vi "GUI_Scopes_1.0.0.vi"() -> ()   [LabVIEW 2013]
uses:
  <vilib>/Utility/miscctls.llb/LVRectTypeDef.ctl
  Device Drivers/shared/scopeTraceInfo_TypDEf.ctl
  Shared/type definition/trace_TypDef.ctl
  Device Drivers/PXIdigitizer/coupling_Enum_TypDef.ctl
  Device Drivers/PXIdigitizer/impedance_Enum_TypDEf.ctl
panel:
  out "ratio(h)":bool=TRUE
  out "fixsize":bool
  out "Change Ratio":cluster{"X":sgl, "Y":sgl}={"X"=1.6671598, "Y"=0.6151203}
  out "old Panel Bounds":T1={"Left"=105, "Top"=80, "Right"=781, "Bottom"=662}
  in  "shotnumber":i32=354
  in  "Save":bool
  in  "Trigger":bool
  in  "Trig.Delay":dbl
  out "error (h)":bool
  in  "impedance":T2
  in  "Channel":enum16{"Channel1", "Channel2"}(ring)
  in  "probeattenuation":dbl
  out "Channel Selector":string
  in  "channelenabled":enum16{"off", "on"}(ring)
  in  "coupling":T3
  in  "offset":dbl=0.52
  in  "verticalrange":dbl
  in  "scopeTrace.Channel1":T4
  in  "scopeTrace.Channel2":T4
  out "Device Name (h)":string="FakeCam1"
  in  "Main Tap":enum32{"IMAQ", "Network", "Internal", "Array"}(tab)
  out "XY Graph":cluster{dbl, dbl}[](graph)
  out "output waveform":waveform(dbl)[](graph)
  out "local Port":u16=65401
  out "Remote Host":string="192.168.10.157"
  out "port or service name":u16=65400
  in  "timeout ms (slow resp)":i32=500
  in  "reset":bool
  out "image con closed":bool=TRUE
  out "image \nconnection":bool
  out "image con closed 2":bool=TRUE
  out "image \nconnection 2":bool
  out "All Devices (h)":string[](array[string])
  out "fast ID (h)":refnum<k16>
  out "slow ID (h)":refnum<k16>
  out "error out":errorcluster
  out "data connection ID (h)":refnum<k5>
  out "connections (hidden)":variant[](array[variant])=[variant(refnum<k16> refnum), variant(refnum<k16> refnum)]
  in  "time to wait (main loop)":i32=10
  in  "Data String":string="exposure,0.520000\r\ntrigger,off\r\nsave,off\r\ngain,0.000000\r\n"
  out "data out":string="Cam1>>ScanStart>>no error,>>"
  in  "send":bool
  in  "send command":string="ScanStart>>Cam1only.txt"
  out "error 2":bool
  out "error message 2":string
  in  "Local Saving Path":path
  out "stop":bool
  out "error message":string
  out "con ref array":refnum<vi>[](array[refnum])
  out "image connection":bool
  out "data connection ok":bool
  # "Data"
  # "Image"
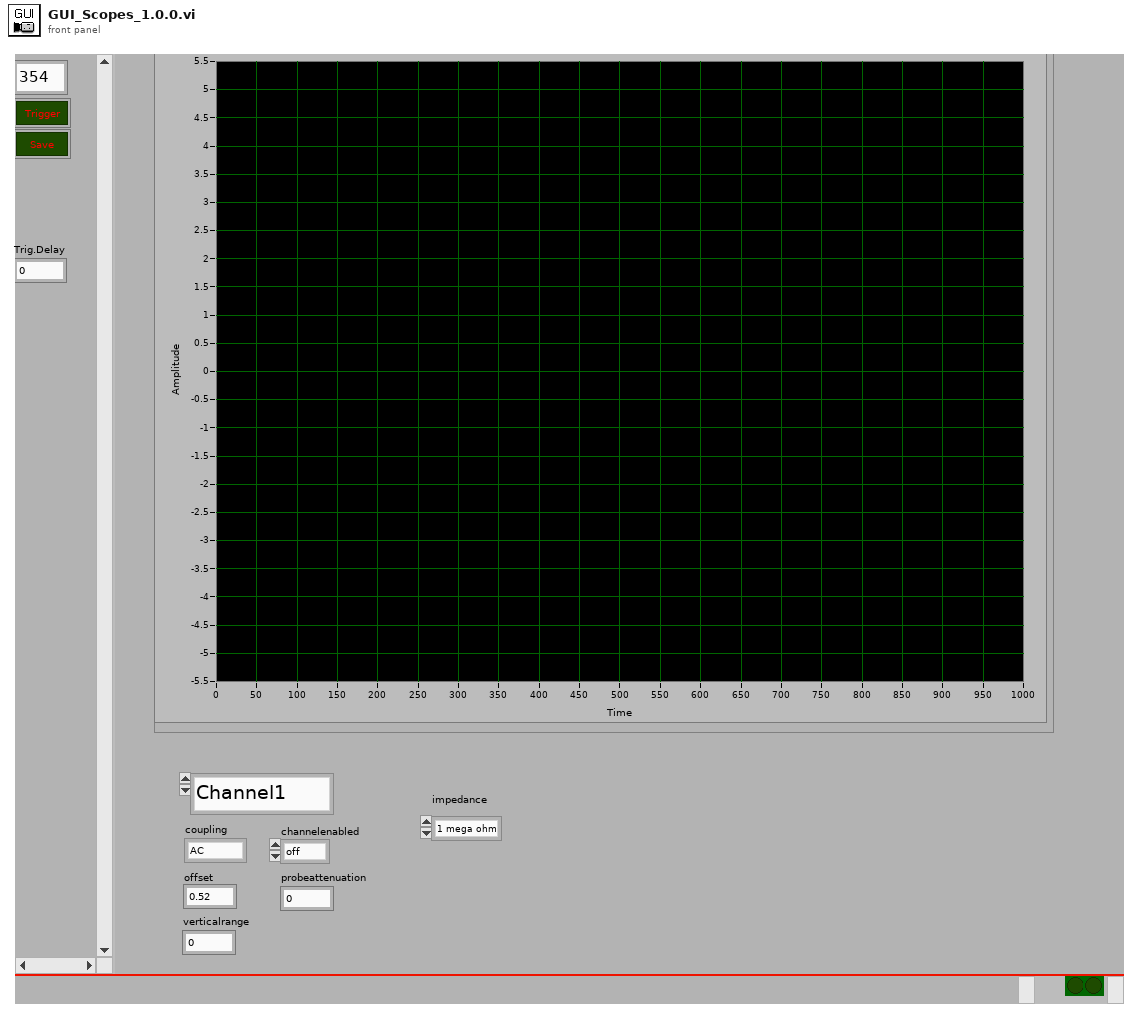
[diagram p1: front panel]
types:
  T1 = typedef "LVRectTypeDef.ctl" = cluster{"Left":i16, "Top":i16, "Right":i16, "Bottom":i16}
  T2 = typedef "impedance_Enum_TypDEf.ctl" = enum16{"1 mega ohm", "<NA>", "50 ohms"}
  T3 = typedef "coupling_Enum_TypDef.ctl" = enum16{"AC", "DC", "Ground"}
  T4 = typedef "trace_TypDef.ctl" = cluster{"info":T5, "wfm":dbl[]}
  T5 = typedef "scopeTraceInfo_TypDEf.ctl" = cluster{"Name":string, "N":dbl, "t0":dbl, "dt":dbl, "offset":dbl, "gain":dbl, "coupling":string, "impedance":string, "range":dbl}
  T6 = typedef "LVBoundsTypeDef.ctl" = cluster{"Width":u32, "Height":u32}
  T7 = typedef "Type Descriptor__ogtk.ctl" = i16[]
  T8 = typedef "Type Descriptor Enumeration__ogtk.ctl" = enum8{"<Null>", "I8", "I16", "I32", "I64", "U8", "U16", "U32", "U64", "SGL", "DBL", "EXT", "CSG", "CDB", "CXT", "0x0F", "0x10", "0x11", "0x12", "0x13", "0x14", "Enum U8", "Enum U16", "Enum U32", "Enum U64", "SGL PQ", "DBL PQ", "EXT PQ", "CSG PQ", "CDB PQ", "CXT PQ", "0x1F", "0x20", "Boolean", "0x22", "0x23", "0x24", "0x25", "0x26", "0x27", "0x28", "0x29", "0x2A", "0x2B", "0x2C", "0x2D", "0x2E", "0x2F", "String", "0x31", "Path", "Pict", "0x34", "0x35", "0x36", "DAQ", "0x38", "0x39", "0x3A", "0x3B", "0x3C", "0x3D", "0x3E", "0x3F", "Array", "0x41", "0x42", "0x43", "0x44", "0x45", "0x46", "0x47", "0x48", "0x49", "0x4A", "0x4B", "0x4C", "0x4D", "0x4E", "0x4F", "Cluster", "0x51", "0x52", "Variant", "Waveform", "0x55", "0x56", "0x57", "0x58", "0x59", "0x5A", "0x5B", "0x5C", "0x5D", "0x5E", "0x5F", "0x60", "0x61", "0x62", "0x63", "0x64", "0x65", "0x66", "0x67", "0x68", "0x69", "0x6A", "0x6B", "0x6C", "0x6D", "0x6E", "0x6F", "Refnum"}
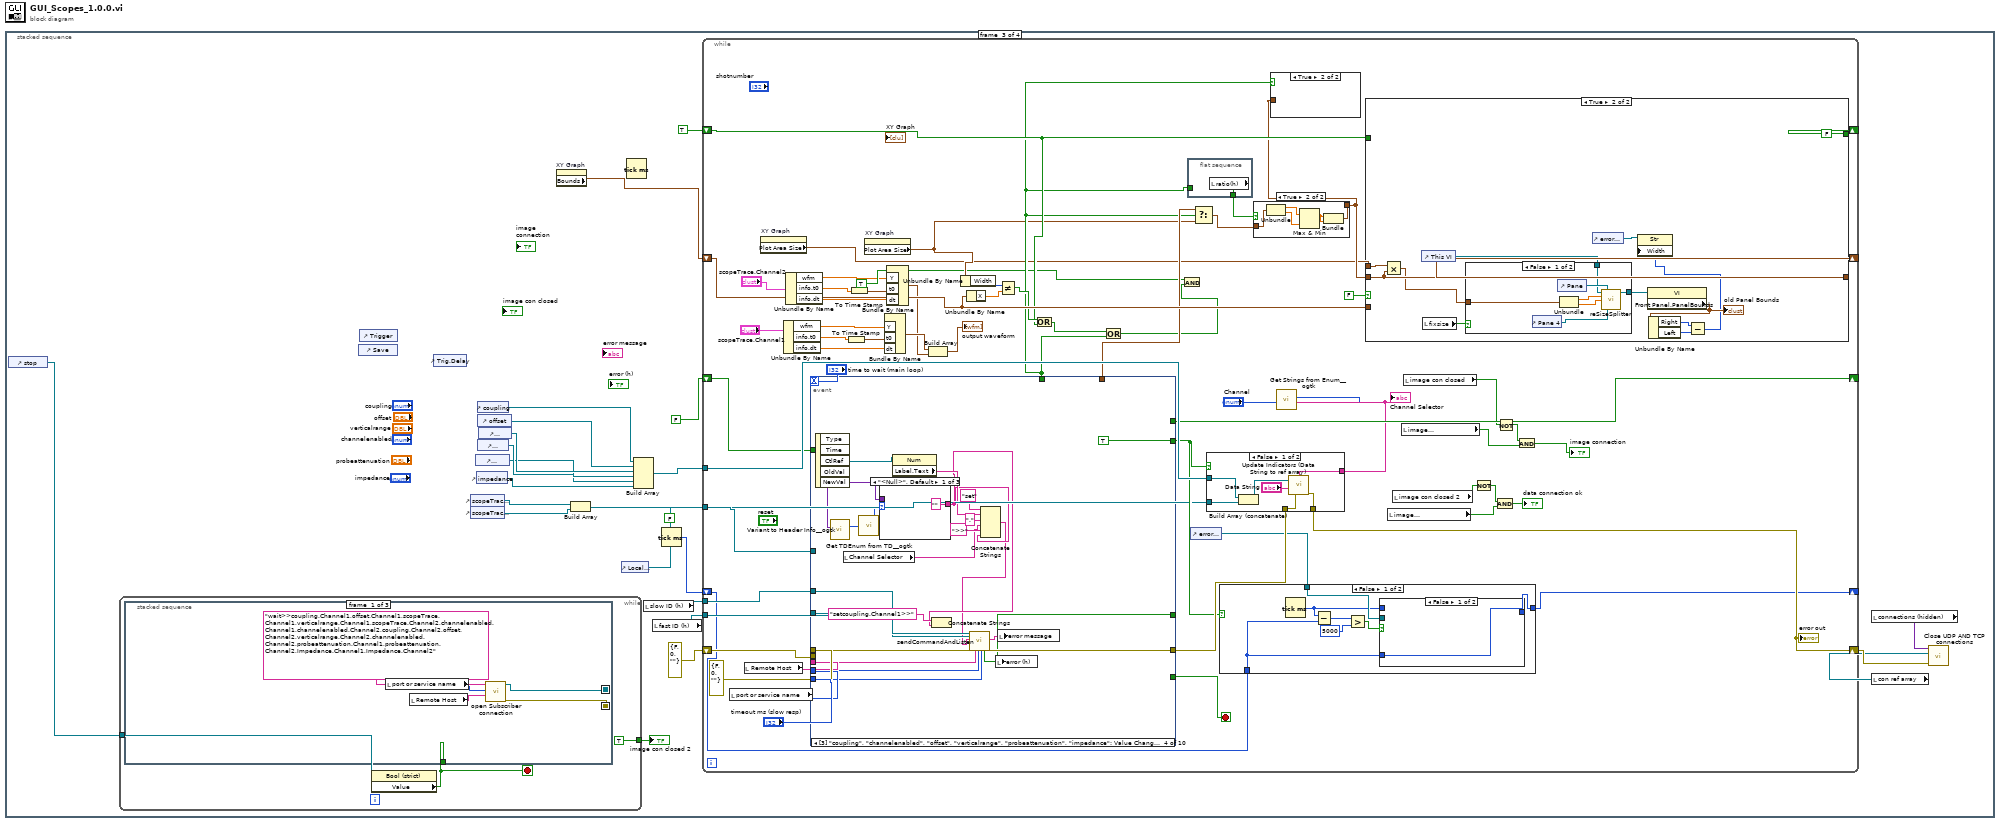
[diagram p0: block diagram]
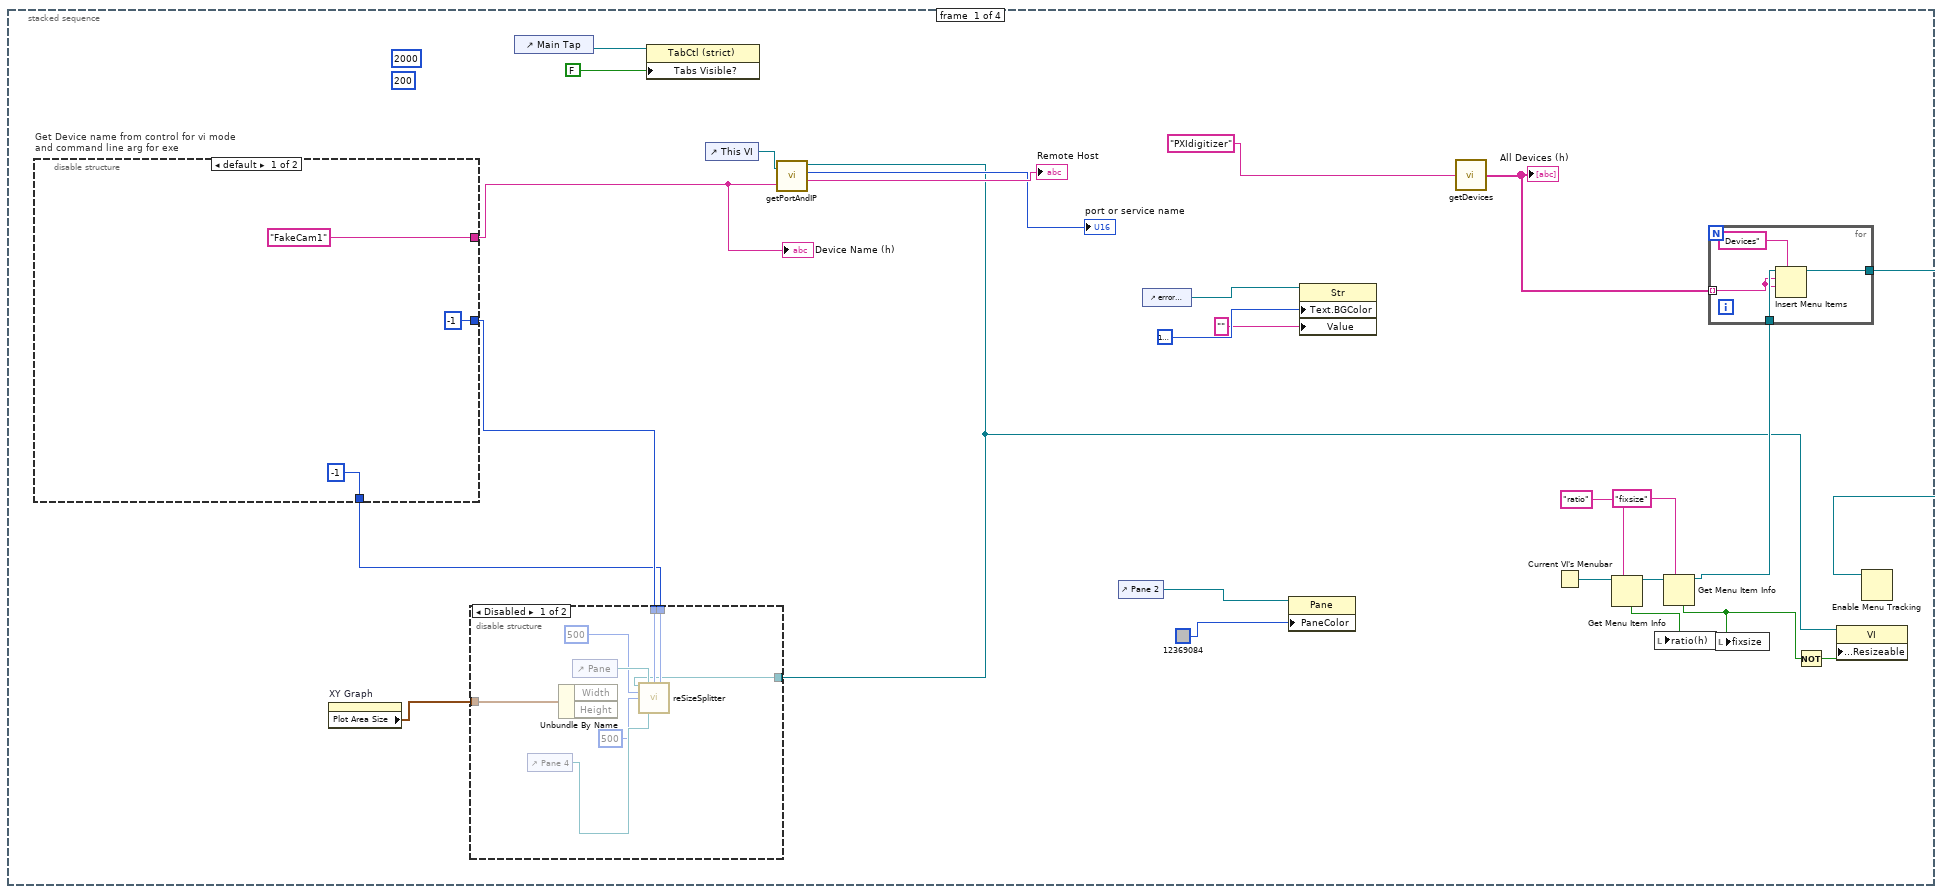
[diagram p2: hidden frame]
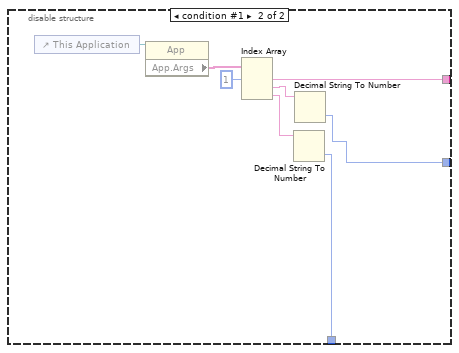
[diagram p4: hidden frame]
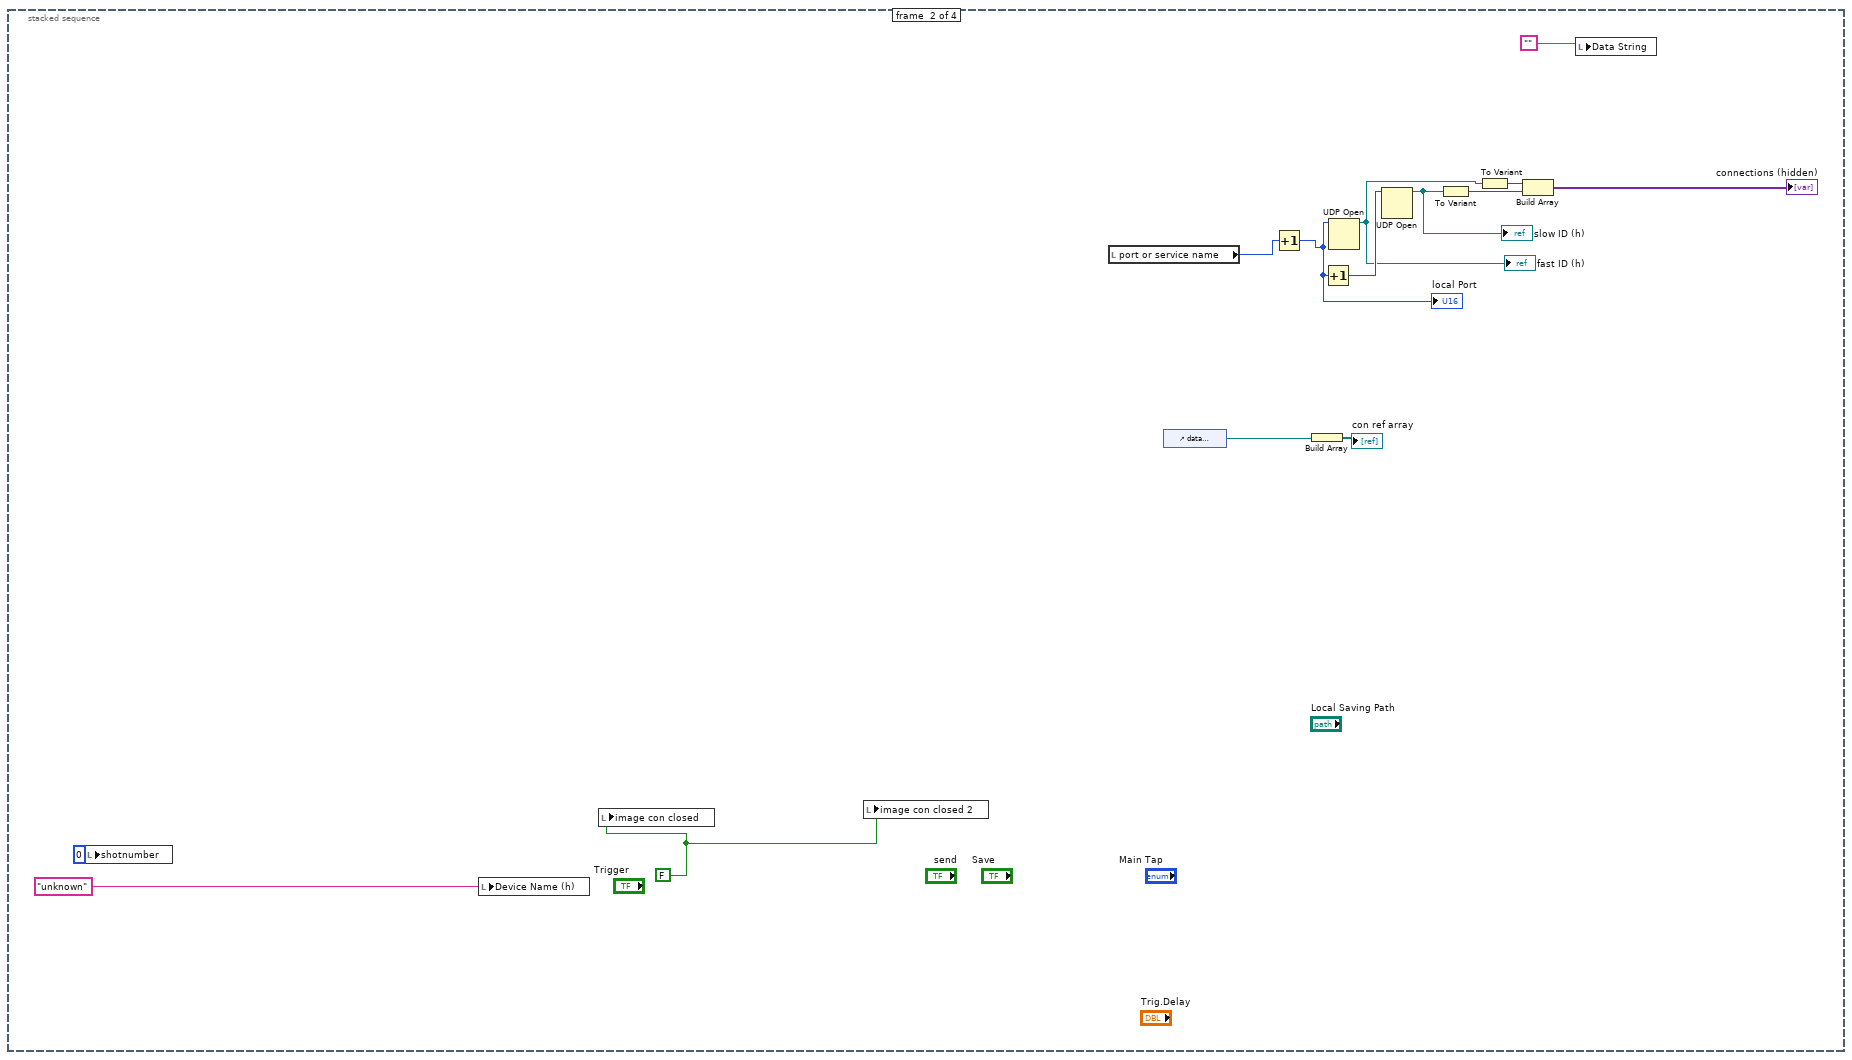
[diagram p5: hidden frame]
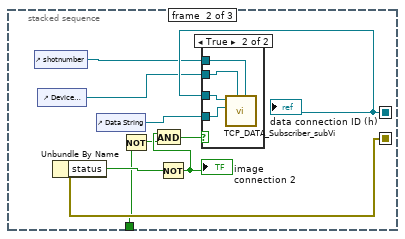
[diagram p6: hidden frame]
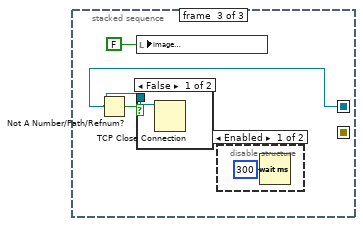
[diagram p8: hidden frame]
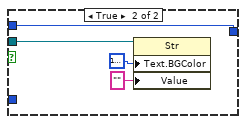
[diagram p11: hidden frame]
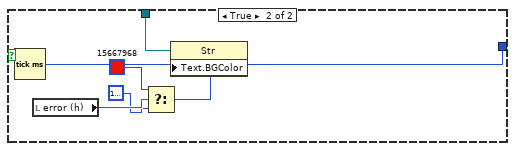
[diagram p12: hidden frame]
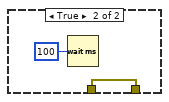
[diagram p17: hidden frame]
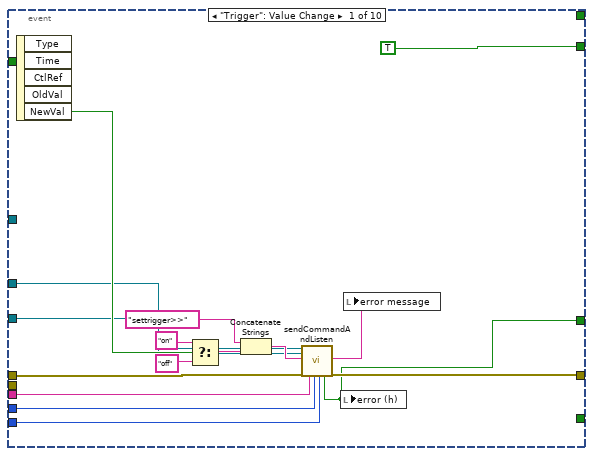
[diagram p18: hidden frame]
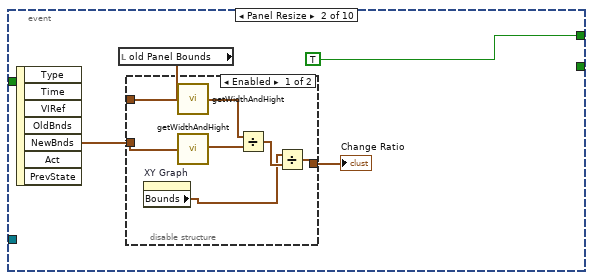
[diagram p19: hidden frame]
diagram:
  n1 = stacked-sequence {
    frame #0 {
      (unwired) i16 2000 ("Left")
      (unwired) i16 200 ("Top")
      n2 = disable-structure "Get Device name from control for vi mode\nand command line arg for exe" shown="default" {
        disable-tunnel: ["FakeCam1" ("Device Name for vi mode") w46] -> w5
        disable-tunnel: [i16 -1 ("left") w43] -> w19
        disable-tunnel: [i16 -1 ("left") w42] -> w18
        frame condition #0 (active) {
        }
        frame condition #1 {
          n3 = control-ref of="This Application"() -> (w49:refnum<vi>)
          n4 = property class="App"(reference=w49) -> ("App.Args"=w48:string[])  [unwired: 1 in, 2 out]
          n5 = Index Array(array=w48, index #1=1 ("index")) -> (element #1=w46:string, element #2=w45:string, element #3=w44:string)  [unwired: 2 in]
          n6 = Decimal String To Number(string=w44) -> (number=w42:i32)  [unwired: 2 in, 1 out]
          n7 = Decimal String To Number(string=w45) -> (number=w43:i32)  [unwired: 2 in, 1 out]
        }
      }
      "Device Name (h)" <- w5
      n8 = property on="XY Graph" class="XYGraph (strict)"() -> ("Plot Area Size"=w1:T6)  [unwired: 2 in, 2 out]
      n9 = control-ref of="Main Tap"() -> (w26:refnum<vi>)
      n10 = property class="TabCtl (strict)"(reference=w26, "Tabs Visible?"=FALSE) -> ()  [unwired: 1 in, 2 out]
      n11 = control-ref of="This VI"() -> (w4:refnum<vi>)
      n12 = call "getPortAndIP.vi"("This Vi"=w4, "Device Name"=w5) -> ("reference out"=w3:refnum<vi>, "port or service name"=→"port or service name":u16, "Remote Host"=→"Remote Host":string)  [unwired: 1 in]
      n13 = disable-structure shown="Disabled" {
        disable-tunnel: w19 -> [w33 _]
        disable-tunnel: w18 -> [w32 _]
        disable-tunnel: w3 -> [w30 _]
        disable-tunnel: w1 -> [w29 _]
        frame Disabled {
          n14 = control-ref of="Pane 4"() -> (w31:refnum<vi>)
          n15 = Unbundle By Name(w29) -> ()  [unwired: 2 out]
          n16 = control-ref of="Pane"() -> (w34:refnum<vi>)
          n17 = call "reSizeSplitter.vi"("this vi"=w30, "pane"=w34, "left"=w33, "top"=w32, "Width"=u32 500, "Height"=u32 500, "pane2"=w31) -> ()  [unwired: 8 in, 1 out]
        }
        frame Enabled {
        }
      }
      n18 = control-ref of="Pane 2"() -> (w12:refnum<vi>)
      n19 = control-ref of="error message"() -> (w14:refnum<vi>)
      n20 = property class="Pane"(reference=w12, "PaneColor"=u32 12369084) -> ()  [unwired: 1 in, 2 out]
      n21 = property class="Str"(reference=w14, "Text.BGColor"=u32 16777238, "Value"="") -> ()  [unwired: 1 in, 2 out]
      n22 = call "getDevices.vi"("Device Class"="PXIdigitizer") -> ("All Devices"=w8:string[])
      "All Devices (h)" <- w8
      n23 = Current VI's Menubar() -> (w23:refnum<k9>)
      n24 = Get Menu Item Info(7:"ratio" ("item tag"), 11:w23) -> (3:w21:refnum<k9>, 4:w22:bool)  [unwired: 1 in, 5 out]
      n25 = local write "ratio(h)"(w22) -> ()
      n26 = Get Menu Item Info(7:"fixsize" ("item tag"), 11:w21) -> (3:w10:refnum<k9>, 4:w16:bool)  [unwired: 1 in, 5 out]
      n27 = for {
        tunnel: w10 -> [w38]
        tunnel: [w37] -> w9
        tunnel: w8 -> [w35] mode=indexing
        n28 = Insert Menu Items(5:"Devices" ("menu tag"), 7:w35, 8:w35, 9:w38) -> (3:w37:refnum<k9>)  [unwired: 2 in, 2 out]
      }
      n29 = local write "fixsize"(w16) -> ()
      n30 = Not(x=w16) -> (.not. x?=w17:bool)
      n31 = property class="VI"(reference=w3, "Front Panel.Resizeable"=w17) -> ()  [unwired: 1 in, 2 out]
      n32 = Enable Menu Tracking(4:w9) -> ()  [unwired: 2 in, 2 out]
    }
    frame #1 {
      w59 = FALSE ("new Device Data")
      n33 = local write "shotnumber"(0 ("shotnumber")) -> ()
      n34 = local write "Device Name (h)"("unknown" ("Device Name")) -> ()
      n35 = local write "image con closed"(w59) -> ()
      n36 = local write "image con closed 2"(w59) -> ()
      n37 = local read "port or service name"() -> (w55:u16)
      n38 = control-ref of="data connection ID (h)"() -> (w63:refnum<vi>)
      n39 = Increment(x=w55) -> (x+1=w52:u16)
      "local Port" <- w52
      n40 = Build Array(w63) -> (→"con ref array":refnum<vi>[])
      n41 = Increment(x=w52) -> (x+1=w56:u16)
      n42 = UDP Open(11:w52) -> (port=w53:refnum<k16>)  [unwired: 4 in, 2 out]
      "fast ID (h)" <- w53
      n43 = UDP Open(11:w56) -> (port=w54:refnum<k16>)  [unwired: 4 in, 2 out]
      "slow ID (h)" <- w54
      n44 = To Variant(anything=w54) -> (Variant=w58:variant)
      n45 = To Variant(anything=w53) -> (Variant=w57:variant)
      n46 = Build Array(w57, w58) -> (→"connections (hidden)":variant[])
      n47 = local write "Data String"("") -> ()
    }
    frame #2 {
      (unwired) FALSE
      n48 = control-ref of="stop"() -> (w79:refnum<vi>)
      n49 = while {
        tunnel: [TRUE] -> w80
        tunnel: w79 -> [w88]
        stop <- w87 stop-if-true
        n50 = property class="Bool (strict)"(reference=w88) -> ("Value"=w87:bool)  [unwired: 1 in, 2 out]
        n51 = stacked-sequence {
          seq-local: [w91 _ _] -> [_ w103 w110]
          seq-local: [w90 _ _] -> [_ w102 _]
          tunnel: w87 -> [_ w96 _]
          frame #0 {
            n52 = local read "port or service name"() -> (w93:u16)
            n53 = local read "Remote Host"() -> (w92:string)
            n54 = call "open Subscriber connection.vi"("Machine"=w92, "Port"=w93, "Subscriber list"="wait>>coupling.Channel1,offset.Channel1,scopeTrace.Channel1,verticalrange.Channel1,scopeTrace.Channel2,channelenabled.Channel1,channelenabled.Channel2,coupling.Channel2,offset.Channel2,verticalrange.Channel2,channelenabled.Channel2,probeattenuation.Channel1,probeattenuation.Channel2,Impedance.Channel1,Impedance.Channel2" ("Subscriber list 2")) -> ("error out"=w90:errorcluster, "connection ID"=w91:refnum<k5>)  [unwired: 3 in]
          }
          frame #1 {
            n55 = control-ref of="shotnumber"() -> (w101:refnum<vi>)
            n56 = control-ref of="Device Name (h)"() -> (w100:refnum<vi>)
            n57 = Unbundle By Name(w102) -> ("status"=w99:bool)
            n58 = control-ref of="Data String"() -> (w104:refnum<vi>)
            n59 = Not(x=w96) -> (.not. x?=w97:bool)
            n60 = Not(x=w99) -> (.not. x?=w98:bool)
            "image \nconnection 2" <- w98
            n61 = And(x=w98, y=w97) -> (x .and. y?=w95:bool)
            n62 = case shown="True" w95 {
              tunnel: w104 -> [_ w108]
              tunnel: w103 -> [_ w107]
              tunnel: w101 -> [_ w106]
              tunnel: w100 -> [_ w105]
              frame False {
              }
              frame True {
                n63 = call "TCP_DATA_Subscriber_subVi.vi"("shot number"=w106, "whatamI"=w105, 10:w108, "connection ID"=w107) -> ()  [unwired: 7 in, 1 out]
              }
            }
            "data connection ID (h)" <- w103
          }
          frame #2 {
            n64 = Not A Number/Path/Refnum?(number/path/refnum=w110) -> (NaN/Path/Refnum?=w111:bool)
            n65 = local write "image \nconnection 2"(FALSE ("status 2")) -> ()
            n66 = case shown="False" w111 {
              tunnel: w110 -> [w113 _]
              frame False {
                n67 = TCP Close Connection(connection ID=w113) -> ()  [unwired: 2 in, 2 out]
              }
              frame True {
              }
            }
            n68 = disable-structure shown="Enabled" {
              frame Enabled {
                n69 = Wait (ms)(milliseconds to wait=u32 300 ("millisecond multiple")) -> ()  [unwired: 1 out]
              }
              frame Disabled {
              }
            }
          }
        }
      }
      "image con closed 2" <- w80
      n70 = control-ref of="Save"() -> ()  [unwired: 1 out]
      n71 = control-ref of="Trigger"() -> ()  [unwired: 1 out]
      n72 = control-ref of="Trig.Delay"() -> ()  [unwired: 1 out]
      n73 = control-ref of="scopeTrace.Channel1"() -> (w68:refnum<vi>)
      n74 = control-ref of="scopeTrace.Channel2"() -> (w67:refnum<vi>)
      n75 = control-ref of="probeattenuation"() -> (w65:refnum<vi>)
      n76 = control-ref of="impedance"() -> (w64:refnum<vi>)
      n77 = control-ref of="coupling"() -> (w71:refnum<vi>)
      n78 = control-ref of="offset"() -> (w72:refnum<vi>)
      n79 = control-ref of="channelenabled"() -> (w69:refnum<vi>)
      n80 = control-ref of="verticalrange"() -> (w70:refnum<vi>)
      n81 = property on="XY Graph" class="XYGraph (strict)"() -> ("Bounds"=w74:T6)  [unwired: 2 in, 2 out]
      n82 = Build Array(w68, w67) -> (w66:refnum<vi>[])
      n83 = control-ref of="Local Saving Path"() -> (w75:refnum<vi>)
      n84 = Tick Count (ms)() -> ()  [unwired: 1 out]
      n85 = Build Array(w71, w72, w70, w69, w65, w64) -> (w73:refnum<vi>[])
      n86 = local read "slow ID (h)"() -> (w84:refnum<k16>)
      n87 = local read "fast ID (h)"() -> (w85:refnum<k16>)
      n88 = Tick Count (ms)() -> (millisecond timer value=w76:u32)
      n89 = while {
        tunnel: w85 -> [w167]
        shift-right: [w164] -> w83
        shift-left: errorcluster {"status"=FALSE, "code"=0, "source"=""} ("error out") -> [w170]
        tunnel: w84 -> [w166]
        tunnel: w73 -> [w172]
        shift-right: [w163] -> _
        shift-left: w74 -> [w162]
        shift-right: [w156] -> _
        shift-left: FALSE -> [w157]
        shift-right: [w155] -> _
        shift-left: TRUE -> [w154]
        shift-right: [w138] -> _
        shift-left: w76 -> [w137]
        tunnel: w75 -> [w134]
        tunnel: w66 -> [w116]
        stop <- w159 stop-if-true
        n90 = local read "port or service name"() -> (w168:u16)
        n91 = local read "Remote Host"() -> (w169:string)
        n92 = property on="XY Graph" class="XYGraph (strict)"() -> ("Plot Area Size"=w132:T6)  [unwired: 2 in, 2 out]
        n93 = Unbundle By Name("scopeTrace.Channel1") -> ("wfm"=w128:dbl[], "info.t0"=w127:dbl, "info.dt"=w125:dbl)
        n94 = Unbundle By Name("scopeTrace.Channel2") -> ("wfm"=w119:dbl[], "info.t0"=w120:dbl, "info.dt"=w122:dbl)
        n95 = event shown="[3] \"coupling\", \"channelenabled\", \"offset\", \"verticalrange\", \"probeattenuation\", \"impedance\": Value Change" {
          selector: _ -> [_ _ _ _ _ _ _ _ _ _]
          dyn-events: _ -> [_ _ _ _ _ _ _ _ _ _]
          timeout: "time to wait (main loop)" -> [_ _ _ _ _ _ _ _ _ _]
          tunnel: w167 -> [w236 _ _ w281 w298 w314 w326 w343 _ _]
          tunnel: [w234 _ _ w279 w296 w312 w323 w341 w349 _] -> w165
          tunnel: errorcluster {"status"=FALSE, "code"=0, "source"=""} ("error out") -> [w235 _ _ w280 w297 w313 w324 w342 _ _]
          tunnel: w169 -> [w239 _ _ w278 w295 w311 w327 w340 _ _]
          tunnel: w168 -> [w240 _ _ w277 w294 w310 w322 w339 _ _]
          tunnel: "timeout ms (slow resp)" -> [w241 _ _ w276 w293 w309 w321 w338 _ _]
          tunnel: w166 -> [w237 _ _ w282 w299 w315 w325 w344 _ _]
          tunnel: w170 -> [_ _ _ _ _ _ _ _ w349 _]
          tunnel: [TRUE _ _ TRUE TRUE TRUE TRUE TRUE _ _] -> w135
          tunnel: [_ _ _ _ _ _ _ _ _ w355] -> w159
          tunnel: [_ _ _ _ _ _ _ _ w348 w352] -> w147
          tunnel: w157 -> [_ _ _ _ _ _ _ _ w348 _]
          tunnel: [_ TRUE _ _ _ _ _ _ _ _] -> w156
          tunnel: [_ _ _ _ _ _ _ _ w347 _] -> w151
          tunnel: [w231 _ _ w273 w290 w304 w318 w334 _ _] -> _
          tunnel: w134 -> [_ _ _ _ _ _ _ _ _ w350]
          event "Trigger": Value Change {
            n96 = event-data() -> ("NewVal"=w246:bool)  [unwired: 1 in, 4 out]
            n97 = Select(t="on", s=w246, f="off") -> (s? t:f=w242:string)
            n98 = Concatenate Strings("settrigger>>" ("data in"), w242) -> (w238:string)
            n99 = call "sendCommandAndListen.vi"(0:w237, 1:w236, "command in"=w238, "error in"=w235, "Remote Host"=w239, "port or service name"=w240, "timeout ms (100)"=w241) -> ("error"=w231:bool, "error message"=w233:string, "error out"=w234:errorcluster)  [unwired: 5 in, 5 out]
            n100 = local write "error (h)"(w231) -> ()
            n101 = local write "error message"(w233) -> ()
          }
          event Panel Resize {
            n102 = event-data() -> ("NewBnds"=w250:T1)  [unwired: 1 in, 6 out]
            n103 = local read "old Panel Bounds"() -> (w248:T1)
            n104 = disable-structure shown="Enabled" {
              disable-tunnel: w250 -> [w257 _]
              disable-tunnel: w248 -> [w253 _]
              disable-tunnel: [w252 _] -> w247
              frame Enabled {
                n105 = property on="XY Graph" class="XYGraph (strict)"() -> ("Bounds"=w251:T6)  [unwired: 2 in, 2 out]
                n106 = call "getWidthAndHight.vi"("OldBnds"=w253) -> ("output cluster"=w256:cluster{"X":sgl, "Y":sgl})
                n107 = call "getWidthAndHight.vi"("OldBnds"=w257) -> ("output cluster"=w255:cluster{"X":sgl, "Y":sgl})
                n108 = Divide(x=w256, y=w255) -> (x/y=w254:cluster{"X":sgl, "Y":sgl})
                n109 = Divide(x=w251, y=w254) -> (x/y=w252:cluster{sgl, sgl})
              }
              frame Disabled {
              }
            }
            "Change Ratio" <- w247
          }
          event "reset": Value Change {
            n110 = event-data() -> ()  [unwired: 1 in, 5 out]
            n111 = flat-sequence {
              frame #0 {
                n112 = local read "con ref array"() -> (w259:refnum<vi>[])
                n113 = call "Close UDP AND TCP connections.vi"("appended array 2"=w259) -> ()  [unwired: 7 in]
              }
              frame #1 {
                n114 = Wait (ms)(milliseconds to wait=u32 1000) -> ()  [unwired: 1 out]
              }
            }
            n115 = local write "reset"(FALSE ("reset")) -> ()
          }
          event "channelenabled", "offset", "verticalrange", "probeattenuation": Value Change {
            n116 = event-data() -> ("CtlRef"=w272:refnum<vi>, "NewVal"=w263:variant)  [unwired: 1 in, 3 out]
            n117 = call <userlib>:"Variant to Header Info__ogtk.vi"("Variant"=w263) -> ("Type Descriptor"=w262:T7)  [unwired: 3 in, 2 out]
            n118 = local read "Channel Selector"() -> (w264:string)
            n119 = call <userlib>:"Get TDEnum from TD__ogtk.vi"("Type Descriptor"=w262) -> ("Type Descriptor Enumeration"=w261:T8)  [unwired: 4 in]
            n120 = case shown="\"<Null>\", Default" w261 {
              tunnel: ["" ("String Value") w285 w286] -> w266
              tunnel: w263 -> [_ w284 w289]
              frame "<Null>", Default {
              }
              frame "Enum U16" {
                n121 = call <userlib>:"Get Strings from Enum__ogtk.vi"("Enum"=w284) -> ("String Value"=w285:string)  [unwired: 7 in, 3 out]
              }
              frame "I8".."CXT" {
                n122 = Variant To Data(type=0.0, Variant=w289) -> (data=w287:dbl)  [unwired: 1 in, 1 out]
                n123 = Number To Fractional String(number=w287) -> (F-format string=w286:string)  [unwired: 3 in]
              }
            }
            n124 = property class="Num"(reference=w272) -> ("Label.Text"=w270:string)  [unwired: 1 in, 2 out]
            n125 = Concatenate Strings("setcoupling.Channel1>>" ("data in"), w266) -> ()  [unwired: 1 out]
            n126 = Concatenate Strings("set", w270, "." ("string"), w264, ">>" ("string"), w266) -> (w265:string)
            n127 = call "sendCommandAndListen.vi"(0:w282, 1:w281, "command in"=w265, "error in"=w280, "Remote Host"=w278, "port or service name"=w277, "timeout ms (100)"=w276) -> ("error"=w273:bool, "error message"=w275:string, "error out"=w279:errorcluster)  [unwired: 5 in, 5 out]
            n128 = local write "error (h)"(w273) -> ()
            n129 = local write "error message"(w275) -> ()
          }
          event "Trig.Delay": Value Change {
            n130 = event-data() -> ("NewVal"=w301:dbl)  [unwired: 1 in, 4 out]
            n131 = Number To Fractional String(number=w301) -> (F-format string=w302:string)  [unwired: 3 in]
            n132 = Concatenate Strings("settriggerdelay>>" ("data in"), w302) -> (w300:string)
            n133 = call "sendCommandAndListen.vi"(0:w299, 1:w298, "command in"=w300, "error in"=w297, "Remote Host"=w295, "port or service name"=w294, "timeout ms (100)"=w293) -> ("error"=w290:bool, "error message"=w292:string, "error out"=w296:errorcluster)  [unwired: 5 in, 5 out]
            n134 = local write "error (h)"(w290) -> ()
            n135 = local write "error message"(w292) -> ()
          }
          event "Local Saving Path": Value Change {
            n136 = event-data() -> ("NewVal"=w306:path)  [unwired: 1 in, 4 out]
            n137 = Path To String(path=w306) -> (string=w305:string)
            n138 = Concatenate Strings("setlocalsavingpath>>" ("data in"), w305) -> (w316:string)
            n139 = call "sendCommandAndListen.vi"(0:w315, 1:w314, "command in"=w316, "error in"=w313, "Remote Host"=w311, "port or service name"=w310, "timeout ms (100)"=w309) -> ("error"=w304:bool, "error message"=w308:string, "error out"=w312:errorcluster)  [unwired: 5 in, 5 out]
            n140 = local write "error (h)"(w304) -> ()
            n141 = local write "error message"(w308) -> ()
          }
          event "Save": Value Change {
            n142 = event-data() -> ("NewVal"=w333:bool)  [unwired: 1 in, 4 out]
            n143 = Select(t="on", s=w333, f="off") -> (s? t:f=w329:string)
            n144 = Concatenate Strings("setsave>>" ("data in"), w329) -> (w328:string)
            n145 = call "sendCommandAndListen.vi"(0:w325, 1:w326, "command in"=w328, "error in"=w324, "Remote Host"=w327, "port or service name"=w322, "timeout ms (100)"=w321) -> ("error"=w318:bool, "error message"=w320:string, "error out"=w323:errorcluster)  [unwired: 5 in, 5 out]
            n146 = local write "error (h)"(w318) -> ()
            n147 = local write "error message"(w320) -> ()
          }
          event "send": Value Change {
            n148 = event-data() -> ()  [unwired: 1 in, 5 out]
            n149 = local write "send"(FALSE ("sent")) -> ()
            n150 = call "sendCommandAndListen.vi"(0:w344, 1:w343, "command in"="send command", "error in"=w342, "Remote Host"=w340, "port or service name"=w339, "timeout ms (100)"=w338) -> ("error"=w334:bool, "error message"=→"error message 2":string, "data out"=→"data out":string, "error out"=w341:errorcluster)  [unwired: 5 in, 4 out]
            "error 2" <- w334
          }
          event Timeout {
            n151 = event-data() -> ()  [unwired: 1 in, 2 out]
            n152 = local read "Change Ratio"() -> (w347:cluster{"X":sgl, "Y":sgl})
          }
          event Menu Selection (User) {
            n153 = event-data() -> ("MenuRef"=w351:refnum<k9>, "ItemTag"=w353:string)  [unwired: 1 in, 3 out]
            n154 = Equal?(x="Exit", y=w353) -> (x = y?=w355:bool)
            "stop" <- w355
            n155 = property on="Main Tap" class="TabCtl (strict)"() -> ("Value"=w357:enum32{"IMAQ", "Network", "Internal", "Array"})  [unwired: 2 in, 2 out]
            n156 = case shown="False" w355 {
              tunnel: w357 -> [w410 _]
              tunnel: w353 -> [w409 _]
              tunnel: [w406 errorcluster {"status"=FALSE, "code"=0, "source"=""} ("error out")] -> w354
              frame False {
                n157 = call <userlib>:"Set Enum String Value__ogtk.vi"("String Value"=w409, "Default Enum Value"=w410) -> ("error out"=w408:errorcluster, "Enum"=w412:variant)  [unwired: 8 in]
                n158 = Variant To Data(error in=w408, type=w410, Variant=w412) -> (data=w411:enum32{"IMAQ", "Network", "Internal", "Array"}, error out=w407:errorcluster)
                n159 = property on="Main Tap" class="TabCtl (strict)"(error in=w407, "Value"=w411) -> (error out=w406:errorcluster)  [unwired: 1 in, 1 out]
              }
              frame True {
              }
            }
            n160 = case shown="Error" w354 {
              tunnel: w351 -> [_ w362]
              tunnel: w353 -> [_ w366]
              tunnel: [_ w367] -> w352
              tunnel: w350 -> [_ w360]
              frame No Error {
              }
              frame Error {
                n161 = local read "All Devices (h)"() -> (w364:string[])
                n162 = Get Menu Item Info(7:w366, 11:w362) -> (0:w363:errorcluster, 2:w369:string, 4:w370:bool)  [unwired: 1 in, 4 out]
                n163 = Not(x=w370) -> (.not. x?=w368:bool)
                n164 = Search 1D Array(1D array=w364, element=w366) -> (index of element=w365:i32)  [unwired: 1 in]
                n165 = Greater Or Equal To 0?(x=w365) -> (x >= 0?=w361:bool)
                n166 = case shown="True" w361 {
                  tunnel: w364 -> [_ w374]
                  tunnel: w363 -> [_ _]
                  tunnel: w362 -> [w371 w373]
                  tunnel: [w371 w372] -> w359
                  frame False {
                  }
                  frame True {
                    n167 = for {
                      tunnel: w374 -> [w378] mode=indexing
                      tunnel: w373 -> [w376]
                      tunnel: [w375] -> w372
                      n168 = Set Menu Item Info(6:FALSE ("checked"), 7:w378, 11:w376) -> (3:w375:refnum<k9>)  [unwired: 4 in, 1 out]
                    }
                  }
                }
                n169 = case shown="\"clear\"" w366 {
                  selector: w366 -> [_ w384 _ _ _ _]
                  tunnel: w368 -> [w379 w382 w393 _ _ _]
                  tunnel: [_ _ TRUE _ _ _] -> w367
                  tunnel: w361 -> [_ w385 _ _ _ _]
                  tunnel: w360 -> [_ _ _ w399 _ _]
                  tunnel: [w379 w383 w393 _ _ _] -> w358
                  frame "fixsize" {
                    n170 = control-ref of="This VI"() -> (w381:refnum<vi>)
                    n171 = Not(x=w379) -> (.not. x?=w380:bool)
                    n172 = property class="VI"(reference=w381, "Front Panel.Resizeable"=w380) -> ()  [unwired: 1 in, 2 out]
                    "fixsize" <- w379
                  }
                  frame Default {
                    n173 = case shown="True" w385 {
                      tunnel: w384 -> [_ w392]
                      tunnel: [_ w386] -> w383
                      tunnel: w382 -> [_ w386]
                      frame False {
                      }
                      frame True {
                        n174 = control-ref of="This VI"() -> (w391:refnum<vi>)
                        n175 = control-ref of="reset"() -> (w388:refnum<vi>)
                        n176 = call "getPortAndIP.vi"("This Vi"=w391, "Device Name"=w392) -> ("port or service name"=w389:u16, "Remote Host"=w390:string)  [unwired: 1 in, 1 out]
                        n177 = local write "port or service name"(w389) -> ()
                        n178 = local write "Remote Host"(w390) -> ()
                        n179 = property class="Bool (strict)"(reference=w388, "Val(Sgnl)"=TRUE ("Value (Signaling)")) -> ()  [unwired: 1 in, 2 out]
                      }
                    }
                  }
                  frame "ratio" {
                    "ratio(h)" <- w393
                  }
                  frame "Local Saving Path" {
                    n180 = property class="Path"(reference=w399) -> (reference out=w397:refnum<vi>, "Value"=w398:path)  [unwired: 1 in, 1 out]
                    n181 = call "changePath.vi"("Local Saving in (h)"=w398) -> ("change (h)"=w396:bool, "Local Saving out (h)"=w395:path)  [unwired: 9 in]
                    n182 = case shown="True" w396 {
                      tunnel: w397 -> [_ w401]
                      tunnel: w395 -> [_ w400]
                      frame False {
                      }
                      frame True {
                        n183 = property class="Path"(reference=w401, "Val(Sgnl)"=w400) -> ()  [unwired: 1 in, 2 out]
                      }
                    }
                  }
                  frame "reset" {
                    n184 = control-ref of="reset"() -> (w403:refnum<vi>)
                    n185 = property class="Bool (strict)"(reference=w403, "Val(Sgnl)"=TRUE ("Value (Signaling)")) -> ()  [unwired: 1 in, 2 out]
                  }
                  frame "clear" {
                    n186 = control-ref of="reset"() -> (w405:refnum<vi>)
                    n187 = property class="Bool (strict)"(reference=w405, "Val(Sgnl)"=TRUE ("Value (Signaling)")) -> ()  [unwired: 1 in, 2 out]
                  }
                }
                n188 = Set Menu Item Info(6:w358, 7:w366, 10:w369, 11:w359) -> ()  [unwired: 3 in, 2 out]
              }
            }
          }
        }
        n189 = To Time Stamp(1:w127) -> (0:w126:timestamp)
        n190 = To Time Stamp(1:w120) -> (0:w121:timestamp)
        n191 = property on="XY Graph" class="XYGraph (strict)"() -> ("Plot Area Size"=w133:T6)  [unwired: 2 in, 2 out]
        n192 = Bundle By Name("Y"=w128, "t0"=w126, "dt"=w125) -> (w124:waveform(dbl))  [unwired: 1 in]
        n193 = Bundle By Name("Y"=w119, "t0"=w121, "dt"=w122) -> (w117:waveform(dbl))  [unwired: 1 in]
        n194 = Build Array(w124, w117) -> (→"output waveform":waveform(dbl)[])
        n195 = Unbundle By Name(w133) -> ("Width"=w161:u32)
        n196 = Unbundle By Name(w162) -> ("X"=w160:sgl)
        n197 = Not Equal?(x=w161, y=w160) -> (x != y?=w158:bool)
        n198 = Or(x=w158, y=w154) -> (x .or. y?=w153:bool)
        n199 = Or(x=w153, y=w147) -> (x .or. y?=w148:bool)
        n200 = And(x=TRUE, y=w148) -> ()  [unwired: 1 out]
        n201 = flat-sequence {
          tunnel: [w193] -> w152
          tunnel: w147 -> [_]
          frame #0 {
            n202 = local read "ratio(h)"() -> (w193:bool)
          }
        }
        n203 = control-ref of="error message"() -> (w136:refnum<vi>)
        n204 = Select(t=w151, s=w147, f=w133) -> (s? t:f=w150:cluster{"X":sgl, "Y":sgl})
        n205 = case shown="False" w135 {
          tunnel: [w176 w192] -> w138
          tunnel: w137 -> [w175 _]
          tunnel: w136 -> [w178 w191]
          frame False {
            n206 = Tick Count (ms)() -> (millisecond timer value=w177:u32)
            n207 = Subtract(x=w177, y=w175) -> (x-y=w181:u32)
            n208 = Greater?(x=w181, y=u32 5000) -> (0:w179:bool)
            n209 = case shown="False" w179 {
              tunnel: w178 -> [_ w186]
              tunnel: w177 -> [_ w183]
              tunnel: [w182 w183] -> w176
              tunnel: w175 -> [w182 _]
              frame False {
              }
              frame True {
                n210 = property class="Str"(reference=w186, "Text.BGColor"=u32 16777238, "Value"="") -> ()  [unwired: 1 in, 2 out]
              }
            }
          }
          frame True {
            n211 = Tick Count (ms)() -> (millisecond timer value=w192:u32)
            n212 = local read "error (h)"() -> (w190:bool)
            n213 = Select(t=u32 15667968, s=w190, f=u32 16777238) -> (s? t:f=w187:u32)
            n214 = property class="Str"(reference=w191, "Text.BGColor"=w187) -> ()  [unwired: 1 in, 2 out]
          }
        }
        n215 = case shown="True" w152 {
          tunnel: w150 -> [w194 w196]
          tunnel: [w194 w195] -> w149
          frame False {
          }
          frame True {
            n216 = Unbundle(w196) -> ("X"=w199:sgl, "Y"=w198:sgl)
            n217 = Max & Min(x=w199, y=w198) -> (max(x,y)=w197:sgl)  [unwired: 1 out]
            n218 = Bundle(w197, w197) -> (w195:cluster{sgl, sgl})  [unwired: 1 in]
          }
        }
        n219 = case shown="True" w147 {
          tunnel: w149 -> [_ _]
          frame False {
          }
          frame True {
          }
        }
        n220 = call <userlib>:"Get Strings from Enum__ogtk.vi"("Enum"="Channel") -> ("String Value"=w115:string)  [unwired: 7 in, 3 out]
        "Channel Selector" <- w115
        n221 = case shown="False" w135 {
          tunnel: w172 -> [w224 _]
          tunnel: w165 -> [w227 w230]
          tunnel: [w226 w230] -> w164
          tunnel: w116 -> [w225 _]
          tunnel: w115 -> [w222 _]
          frame False {
            n222 = Build Array (concatenate)(w224, w225) -> (w223:refnum<vi>[])
            n223 = call "Update Indicators (Data String to ref array).vi"("Array"=w223, "Active Channel"=w222, "Data String"="Data String", 12:w227) -> ("error out"=w226:errorcluster)  [unwired: 10 in, 1 out]
          }
          frame True {
            n224 = Wait (ms)(milliseconds to wait=u32 100) -> ()  [unwired: 1 out]
          }
        }
        "error out" <- w164
        n225 = case shown="True" FALSE {
          tunnel: w149 -> [_ w212]
          tunnel: [w201 w212] -> w163
          tunnel: w162 -> [w201 _]
          tunnel: w132 -> [_ w213]
          tunnel: w154 -> [w200 _]
          tunnel: [w200 FALSE] -> w155
          frame False {
          }
          frame True {
            n226 = Multiply(x=w213, y=w212) -> (x*y=w211:cluster{sgl, sgl})
            n227 = control-ref of="This VI"() -> (w209:refnum<vi>)
            n228 = local read "fixsize"() -> (w202:bool)
            n229 = case shown="False" w202 {
              tunnel: w211 -> [w214 _]
              tunnel: w209 -> [w217 w221]
              tunnel: [w216 w221] -> w208
              frame False {
                n230 = control-ref of="Pane 4"() -> (w215:refnum<vi>)
                n231 = control-ref of="Pane"() -> (w218:refnum<vi>)
                n232 = Unbundle(w214) -> (w219:sgl, w220:sgl)
                n233 = call "reSizeSplitter.vi"("this vi"=w217, "pane"=w218, "Width"=w219, "Height"=w220, "pane2"=w215) -> ("reference out"=w216:refnum<vi>)  [unwired: 10 in]
              }
              frame True {
              }
            }
            n234 = control-ref of="error message"() -> (w210:refnum<vi>)
            n235 = property class="VI"(reference=w208) -> ("Front Panel.PanelBounds"=w207:T1)  [unwired: 1 in, 2 out]
            "old Panel Bounds" <- w207
            n236 = Unbundle By Name(w207) -> ("Right"=w206:i16, "Left"=w205:i16)
            n237 = Subtract(x=w206, y=w205) -> (x-y=w204:i16)
            n238 = property class="Str"(reference=w210, "Width"=w204) -> ()  [unwired: 1 in, 2 out]
          }
        }
        n239 = local read "image \nconnection 2"() -> (w144:bool)
        n240 = local read "image con closed 2"() -> (w146:bool)
        n241 = local read "image \nconnection"() -> (w140:bool)
        n242 = local read "image con closed"() -> (w141:bool)
        n243 = Not(x=w146) -> (.not. x?=w145:bool)
        n244 = And(x=w145, y=w144) -> (x .and. y?=→"data connection ok":bool)
        n245 = Not(x=w141) -> (.not. x?=w142:bool)
        n246 = And(x=w142, y=w140) -> (x .and. y?=→"image connection":bool)
      }
      n247 = local read "connections (hidden)"() -> (w81:variant[])
      n248 = local read "con ref array"() -> (w82:refnum<vi>[])
      n249 = call "Close UDP AND TCP connections.vi"("error in"=w83, "appended array 2"=w82, "appended array"=w81) -> ()  [unwired: 5 in]
    }
    frame #3 {
      n250 = flat-sequence {
        frame #0 {
          n251 = Wait (ms)(milliseconds to wait=u32 0) -> ()  [unwired: 1 out]
        }
        frame #1 {
          n252 = local write "stop"(FALSE ("stop")) -> ()
        }
        frame #2 {
          n253 = control-ref of="This VI"() -> (w421:refnum<vi>)
          n254 = case shown="True" FALSE {
            tunnel: w421 -> [w422 w425]
            tunnel: [w422 w423] -> w420
            frame False {
            }
            frame True {
              n255 = property class="VI" props=["Front Panel.Open"](reference=w425) -> (reference out=w424:refnum<vi>)  [unwired: 1 in, 2 out]
              n256 = invoke class="VI" method="FP.Close"(reference=w424) -> (reference out=w423:refnum<vi>)  [unwired: 2 in, 2 out]
            }
          }
          n257 = Close Reference(reference=w420) -> ()  [unwired: 1 in, 1 out]
        }
      }
      n258 = control-ref of="Main  Control"() -> (w415:refnum<vi>)
      n259 = property class="TabCtl (strict)"(reference=w415, "Tabs Visible?"=TRUE) -> ()  [unwired: 1 in, 2 out]
      n260 = property class="TabCtl (strict)"(reference=w415, "Tab Location"=enum32{"Top", "Bottom", "Left", "Right"}."Bottom") -> ()  [unwired: 1 in, 2 out]
    }
  }
